vi "仪器版本写入.vi"(8 "error in (no error)":errorcluster caption="错误输入（无错误）", 10 "仪器版本":T1, 11 "SingleStepTestV3 输入":refnum<class "SingleStepTestV3.lvclass">) -> (0 "error out":errorcluster caption="错误输出", 3 "SingleStepTestV3 输出":refnum<class "SingleStepTestV3.lvclass">)   [LabVIEW 2016, in "SingleStepTestV3.lvlib" / "SingleStepTestV3.lvclass"]
uses:
  SingleStepTestV3.lvclass
  SingleStepTestV3.lvclass/SingleStepTestV3.ctl
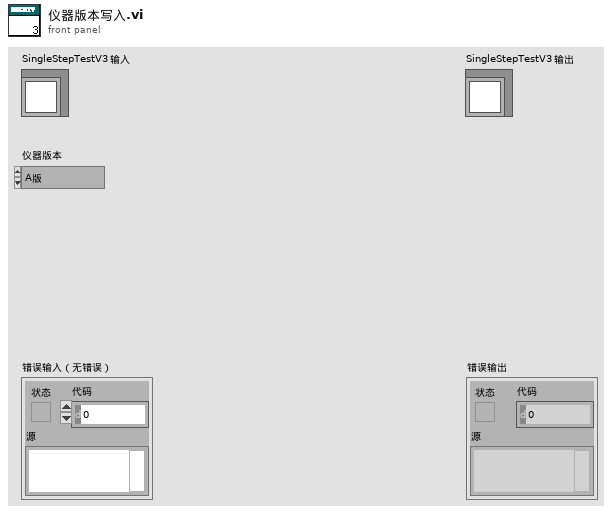
[diagram p1: front panel]
types:
  T1 = typedef "SingleStepTestV3.lvlib/SingleStepTestV3.lvclass/仪器版本.ctl" = enum16{"A版", "B版", "A1版"}
  T2 = typedef "SingleStepTestV3.lvlib/SingleStepTestV3.lvclass/State Data.ctl" = cluster{"data":u16[], "仪器版本":T1}
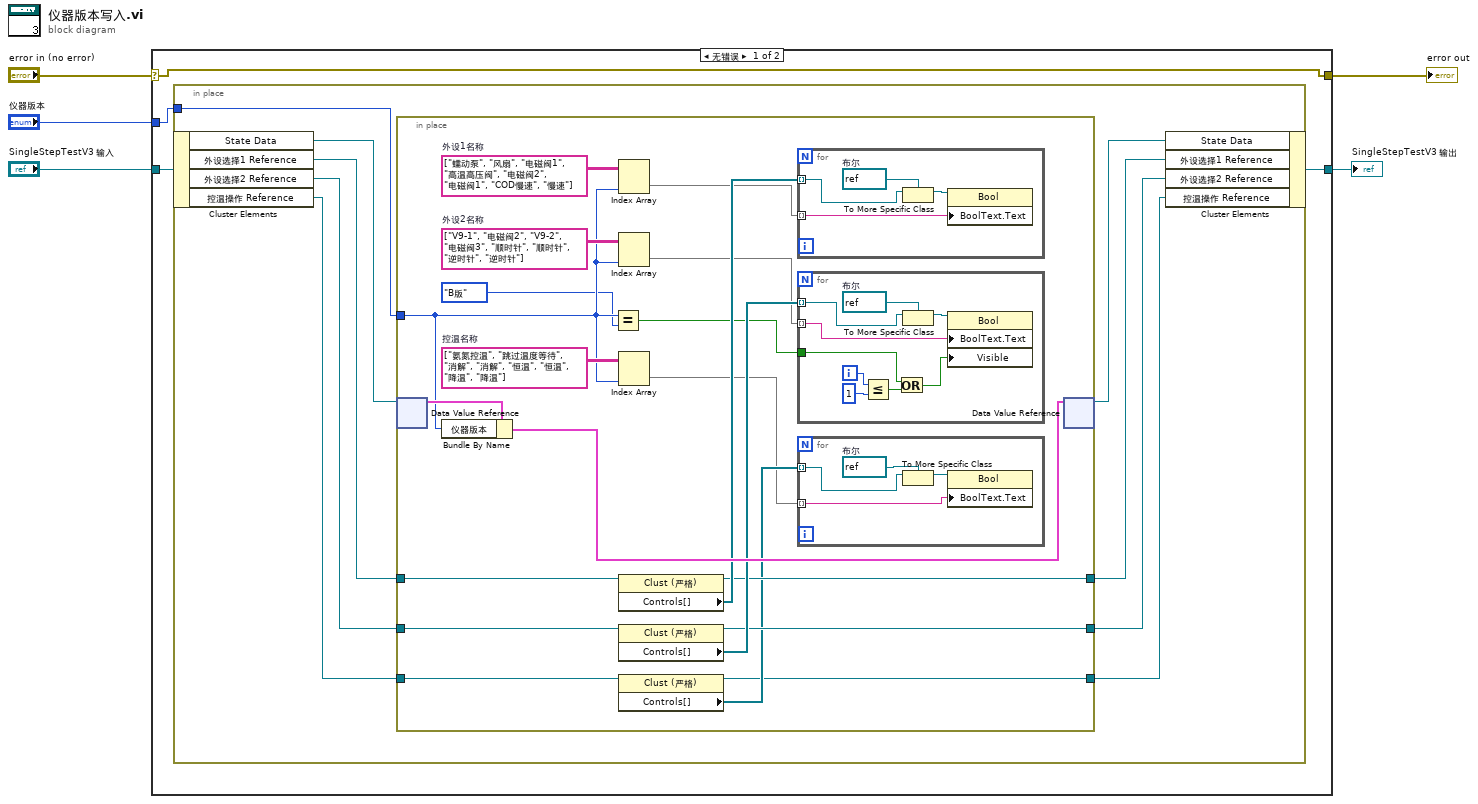
[diagram p0: block diagram]
diagram:
  n1 = case shown="无错误" "error in (no error)" {
    selector: "error in (no error)" -> [w9 w57]
    tunnel: [w9 w57] -> w4
    tunnel: [w7 w56] -> w2
    tunnel: "SingleStepTestV3 输入" -> [w8 w56]
    tunnel: "仪器版本" -> [w6 _]
    frame No Error {
      n2 = in-place {
        in-place-border: w6 -> [w16]
        n3 = in-place-cluster #1(w8) -> ("State Data"=w18:refnum<data-value>, "外设选择1 Reference"=w15:refnum<vi>, "外设选择2 Reference"=w14:refnum<vi>, "控温操作 Reference"=w11:refnum<vi>)
        n4 = in-place {
          in-place-border: w16 -> [w21]
          in-place-border: w15 -> [w36]
          in-place-border: w14 -> [w35]
          in-place-border: [w28] -> w13
          in-place-border: [w27] -> w12
          in-place-border: w11 -> [w26]
          in-place-border: [w22] -> w10
          w24 = string[][] [["氨氮控温", "跳过温度等待"], ["消解", "消解"], ["恒温", "恒温"], ["降温", "降温"]]  # 控温名称
          w30 = string[][] [["V9-1", "电磁阀2"], ["V9-2", "电磁阀3"], ["顺时针", "顺时针"], ["逆时针", "逆时针"]]  # 外设2名称
          w33 = string[][] [["蠕动泵", "风扇"], ["电磁阀1", "高温高压阀"], ["电磁阀2", "电磁阀1"], ["COD慢速", "慢速"]]  # 外设1名称
          n5 = in-place-dvr #2(w18) -> (w38:T2)  [unwired: 1 out]
          n6 = Bundle By Name(cluster=w38, "仪器版本"=w21) -> (w37:T2)
          n7 = Equal?(x=w21, y=仪器版本."B版") -> (x = y?=w19:bool)
          n8 = Index Array(array=w33, index (col)=w21) -> (element=w32:string[])  [unwired: 1 in]
          n9 = Index Array(array=w30, index (col)=w21) -> (element=w29:string[])  [unwired: 1 in]
          n10 = Index Array(array=w24, index (col)=w21) -> (element=w23:string[])  [unwired: 1 in]
          n11 = property class="Clust (严格)"(reference=w36) -> (reference out=w28:refnum<vi>, "Controls[]"=w34:refnum<vi>[])  [unwired: 1 in, 1 out]
          n12 = property class="Clust (严格)"(reference=w35) -> (reference out=w27:refnum<vi>, "Controls[]"=w31:refnum<vi>[])  [unwired: 1 in, 1 out]
          n13 = property class="Clust (严格)"(reference=w26) -> (reference out=w22:refnum<vi>, "Controls[]"=w25:refnum<vi>[])  [unwired: 1 in, 1 out]
          n14 = for {
            tunnel: w34 -> [w55] mode=indexing
            tunnel: w32 -> [w52] mode=indexing
            w53 = refnum<vi> refnum  # 布尔
            n15 = To More Specific Class(target class=w53, reference=w55) -> (specific class reference=w54:refnum<vi>)  [unwired: 1 in, 1 out]
            n16 = property class="Bool"(reference=w54, "BoolText.Text"=w52) -> ()  [unwired: 1 in, 2 out]
          }
          n17 = for {
            tunnel: w31 -> [w51] mode=indexing
            tunnel: w29 -> [w48] mode=indexing
            tunnel: w19 -> [w44]
            i -> [w47]
            w49 = refnum<vi> refnum  # 布尔
            n18 = Less Or Equal?(x=w47, y=1) -> (x <= y?=w45:bool)
            n19 = Or(x=w44, y=w45) -> (x .or. y?=w43:bool)
            n20 = To More Specific Class(target class=w49, reference=w51) -> (specific class reference=w50:refnum<vi>)  [unwired: 1 in, 1 out]
            n21 = property class="Bool"(reference=w50, "BoolText.Text"=w48, "Visible"=w43) -> ()  [unwired: 1 in, 2 out]
          }
          n22 = for {
            tunnel: w25 -> [w42] mode=indexing
            tunnel: w23 -> [w39] mode=indexing
            w40 = refnum<vi> refnum  # 布尔
            n23 = To More Specific Class(target class=w40, reference=w42) -> (specific class reference=w41:refnum<vi>)  [unwired: 1 in, 1 out]
            n24 = property class="Bool"(reference=w41, "BoolText.Text"=w39) -> ()  [unwired: 1 in, 2 out]
          }
          n25 = in-place-dvr #2(w37) -> (w17:refnum<data-value>)  [unwired: 1 out]
        }
        n26 = in-place-cluster #1("State Data"=w17, "外设选择1 Reference"=w13, "外设选择2 Reference"=w12, "控温操作 Reference"=w10) -> (w7:refnum<class "SingleStepTestV3.lvclass">)
      }
    }
    frame Error {
    }
  }
  "error out" <- w4
  "SingleStepTestV3 输出" <- w2
